vi "excelDispatchNew.vi"() -> ()   [LabVIEW 2012]
uses:
  <vilib>/Utility/NIReport.llb/NI_report.lvclass
  Global1.vi
  <vilib>/addons/database/Connection.llb/DB Tools Open Connec (Path).vi
  <vilib>/addons/_office/excel.llb/Excel Get Data (str).vi
  <vilib>/Utility/NIReport.llb/Excel/NI_Excel.lvclass
  <vilib>/addons/_office/NI_ReportGenerationToolkit.lvlib
  <vilib>/addons/database/NI_Database_API.lvlib
panel:
  out "filenames":string[](array[string])
  out "appended path":path
  out "x+y":i32
  out "error out 3":errorcluster
  out "String 2":string
  out "row":i32
  out "error out":errorcluster
  in  "start (0, 0)":cluster{"start row":i32, "start column":i32}
  out "error out 4":errorcluster
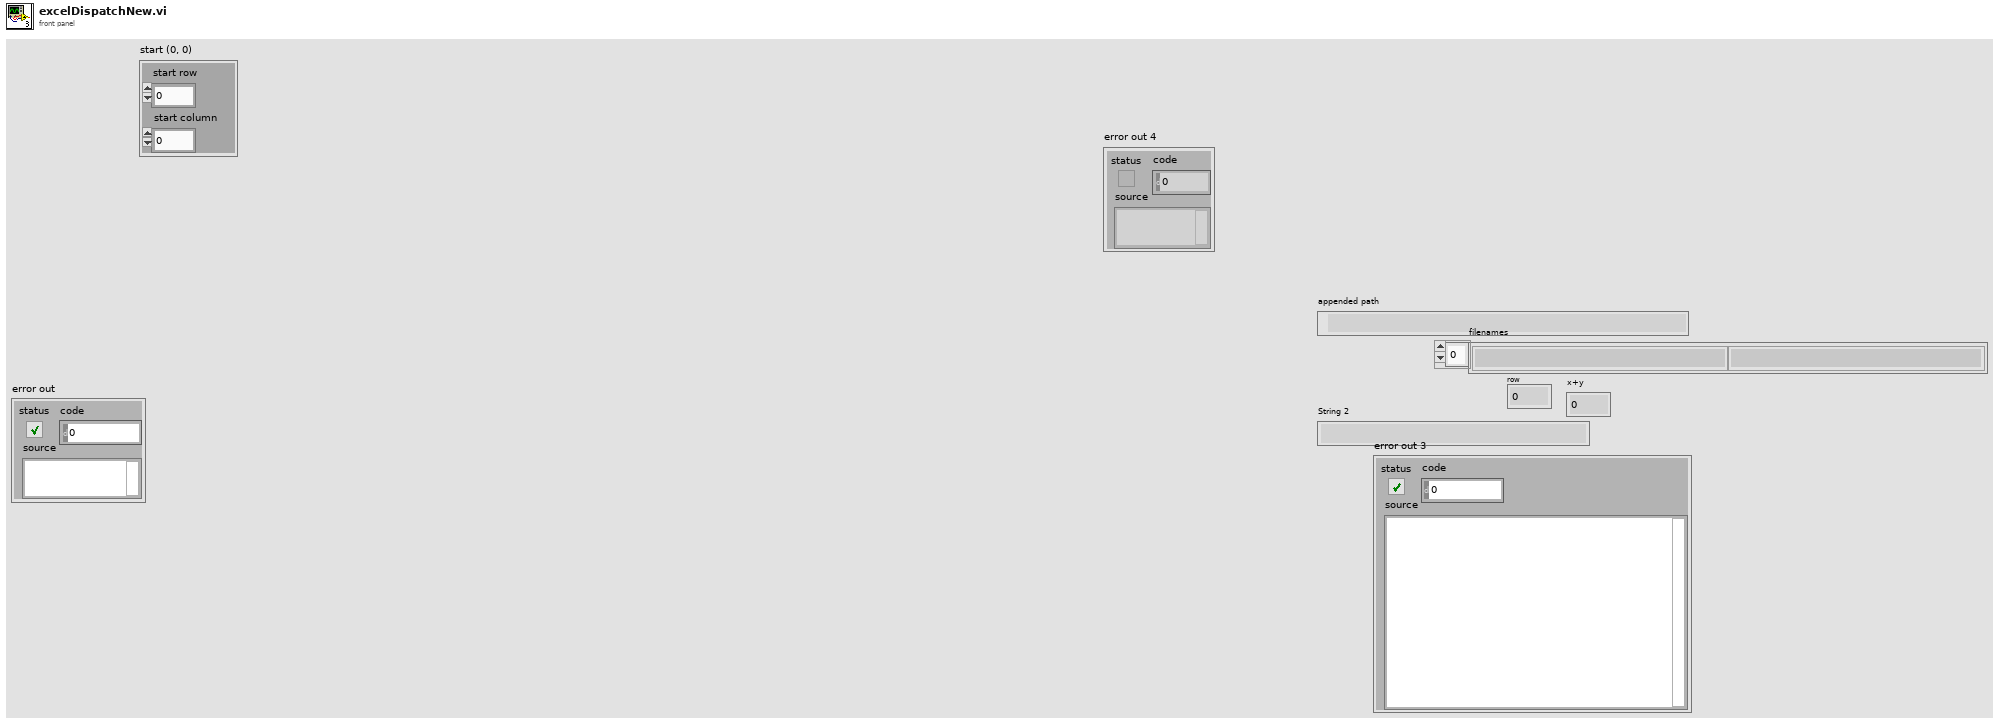
[diagram p1: front panel]
types:
  T1 = enum16{"Standard Report", "HTML", "Word", "Excel"}
  T2 = typedef "NI_Database_API.lvlib/Conn ObjectReference.ctl" = refnum<k1>
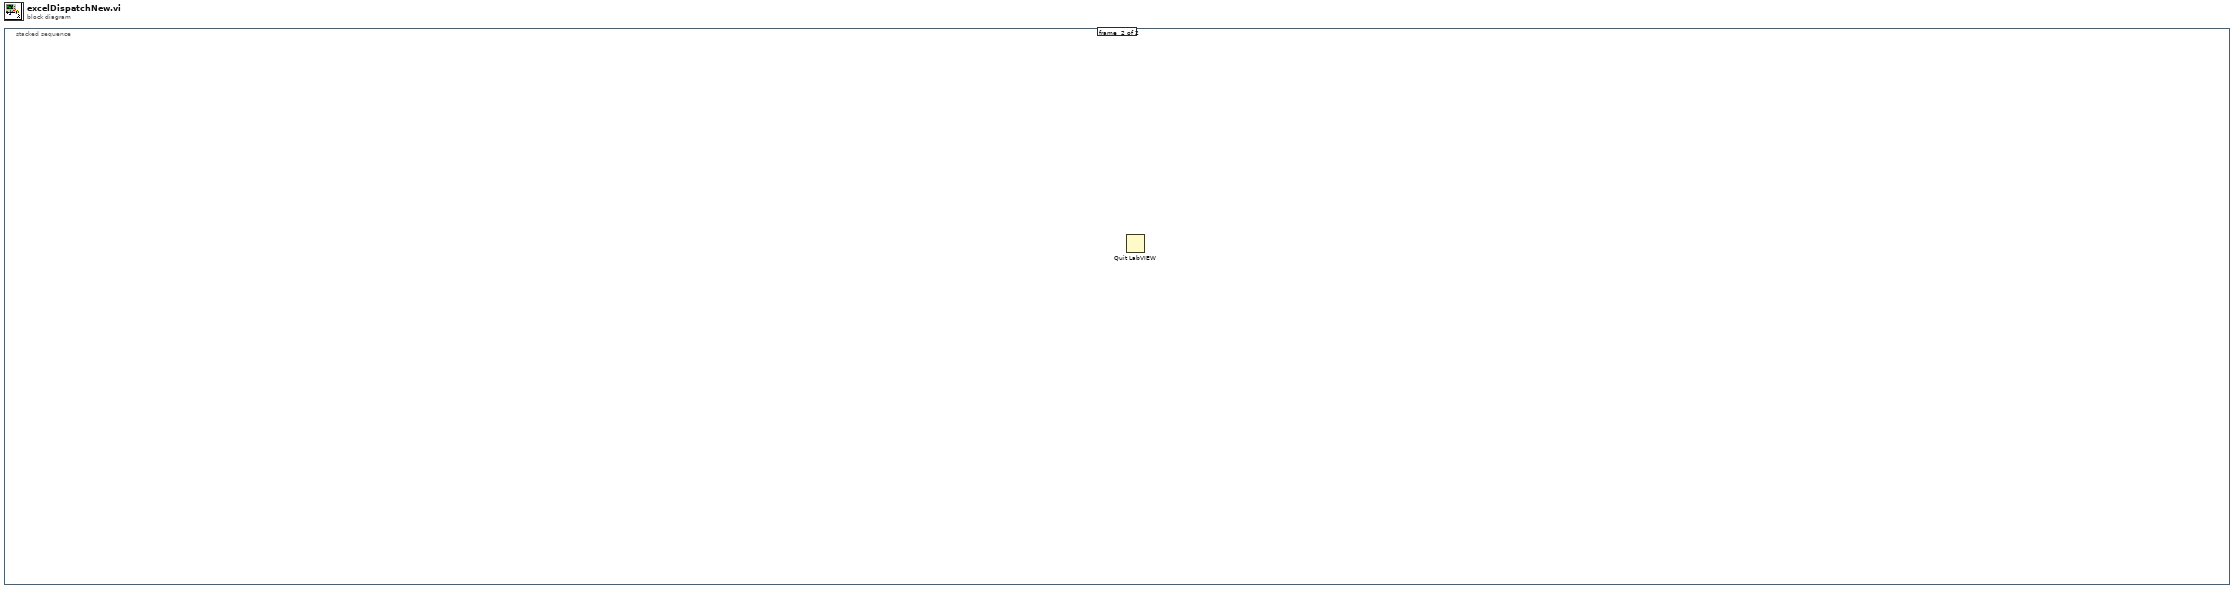
[diagram p0: block diagram]
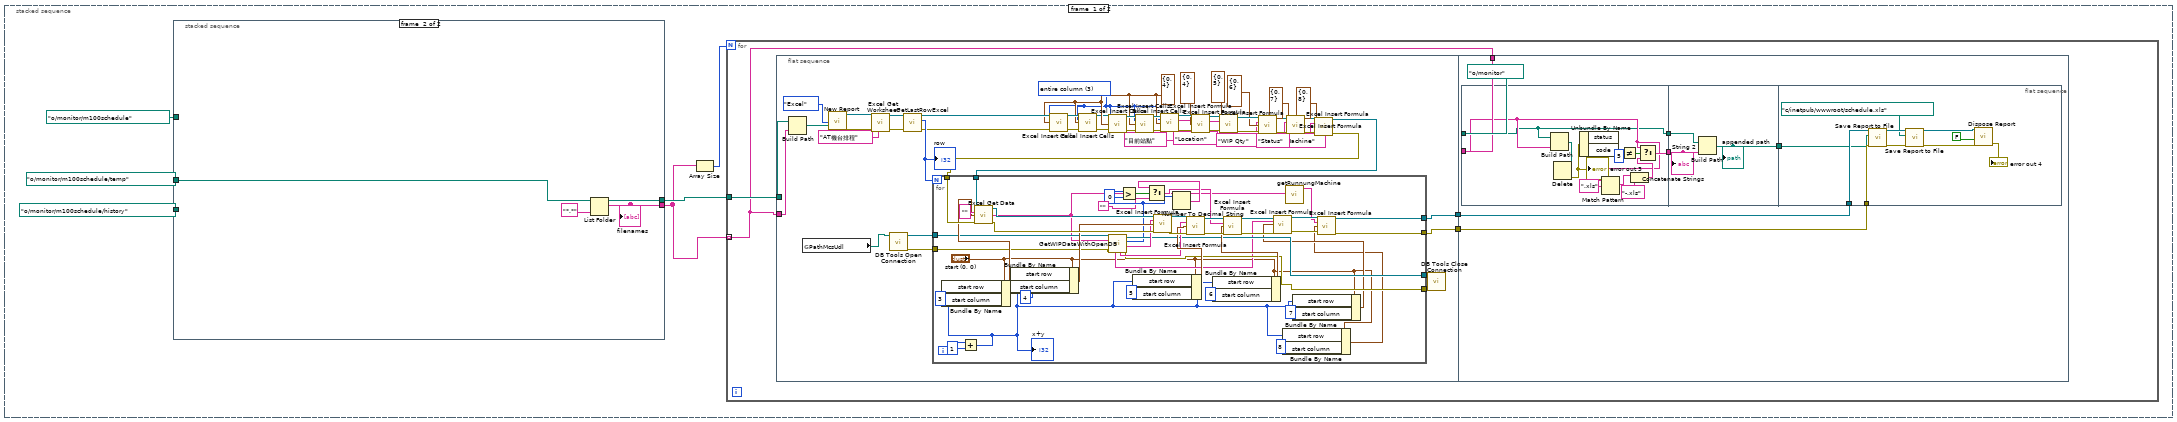
[diagram p2: hidden frame]
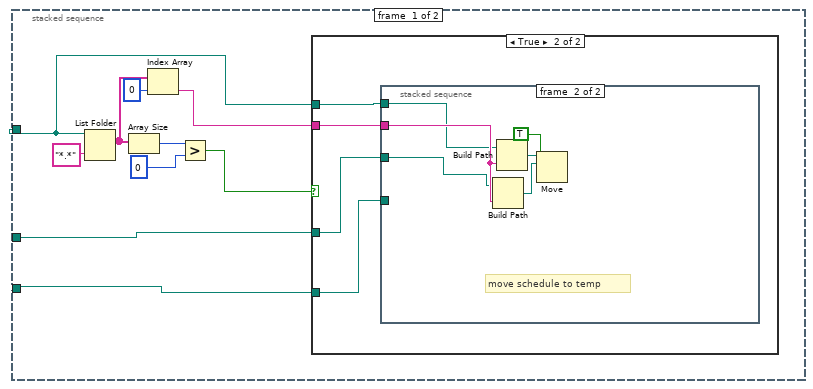
[diagram p3: hidden frame]
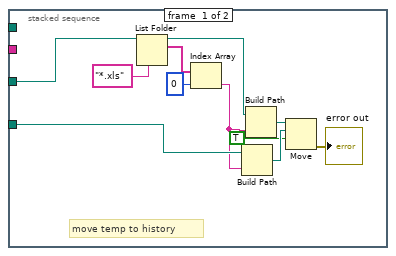
[diagram p5: hidden frame]
diagram:
  n1 = stacked-sequence {
    frame #0 {
      n2 = stacked-sequence {
        tunnel: path "o:/monitor/m100schedule/temp" ("path") -> [w7 w40]
        tunnel: [_ w39] -> w5
        tunnel: path "o:/monitor/m100schedule" ("path") -> [w9 _]
        tunnel: path "o:/monitor/m100schedule/history" ("path") -> [w8 _]
        tunnel: [_ w38] -> w1
        frame #0 {
          n3 = List Folder(path=w9, pattern="*.*") -> (filenames=w13:string[])  [unwired: 2 in, 3 out]
          n4 = Array Size(array=w13) -> (size(s)=w15:i32)
          n5 = Index Array(array=w13, index=0) -> (element=w11:string)
          n6 = Greater?(x=w15, y=0) -> (0:w12:bool)
          n7 = case shown="True" w12 {
            tunnel: w7 -> [_ w20]
            tunnel: w8 -> [_ w19]
            tunnel: w9 -> [_ w18]
            tunnel: w11 -> [_ w17]
            frame False {
            }
            frame True {
              n8 = stacked-sequence {
                tunnel: w20 -> [w27 w33]
                tunnel: w19 -> [w30 _]
                tunnel: w18 -> [_ w34]
                tunnel: w17 -> [_ w35]
                frame #0 {
                  # "move temp to history"
                  n9 = List Folder(path=w27, pattern="*.xls") -> (path out=w25:path, filenames=w24:string[])  [unwired: 2 in, 2 out]
                  n10 = Index Array(array=w24, index=0) -> (element=w22:string)
                  n11 = Build Path(base path=w30, name or relative path=w22) -> (appended path=w29:path)
                  n12 = Build Path(base path=w25, name or relative path=w22) -> (appended path=w31:path)
                  n13 = Move(source path=w31, 9:TRUE ("overwrite (F)"), 10:w29) -> (error out=→"error out":errorcluster)  [unwired: 2 in, 2 out]
                }
                frame #1 {
                  # "move schedule to temp"
                  n14 = Build Path(base path=w33, name or relative path=w35) -> (appended path=w36:path)
                  n15 = Build Path(base path=w34, name or relative path=w35) -> (appended path=w37:path)
                  n16 = Move(source path=w37, 9:TRUE ("overwrite (F)"), 10:w36) -> ()  [unwired: 2 in, 3 out]
                }
              }
            }
          }
        }
        frame #1 {
          n17 = List Folder(path=w40, pattern="*.*") -> (path out=w39:path, filenames=w38:string[])  [unwired: 2 in, 2 out]
          "filenames" <- w38
        }
      }
      n18 = Array Size(array=w1) -> (size(s)=w2:i32)
      n19 = for {
        N: w2 -> [_]
        tunnel: w5 -> [w45]
        tunnel: w1 -> [w42] mode=indexing
        n20 = flat-sequence {
          tunnel: w45 -> [w96]
          tunnel: w42 -> [w95]
          tunnel: [w69] -> w44
          tunnel: [w49] -> w43
          tunnel: w44 -> [w144]
          tunnel: w43 -> [w145]
          tunnel: w42 -> [w146]
          frame #0 {
            w61 = cluster{"row":i32, "column":i32} {"row"=0, "column"=4} ("start (0, 0)")
            w58 = u16 3 items=["shift cells right", "shift cells down", "entire row", "entire column"] ("mode (entire row)")
            n21 = Build Path(base path=w96, name or relative path=w95) -> (appended path=w94:path)
            n22 = global read "Global1.vi" "PathMcsUdl"() -> (w84:path)
            n23 = call <vilib>:"New Report.vi"("report type"=T1."Excel" ("Report Type"), "template (empty)"=w94) -> ("report out"=w92:refnum<class "NI_report.lvclass">, "error out"=w91:errorcluster)  [unwired: 12 in]
            n24 = call <vilib>:"Excel Get Worksheet.vi"("report in"=w92, "error in (no error)"=w91, "name (\"\")"="AT機台排程" ("name (\"\")")) -> ("report out"=w68:refnum<class "NI_report.lvclass">, "error out"=w67:errorcluster)  [unwired: 11 in]
            n25 = call-poly <vilib>:"DB Tools Open Connection.vi"("connection information"=w84) -> ("error out"=w82:errorcluster, "connection reference"=w83:T2)  [unwired: 7 in]
            n26 = call "GetLastRowExcel.vi"("error in (no error)"=w67, "report in"=w68) -> ("error out"=w65:errorcluster, "row"=w66:i32, "report out"=w64:refnum<class "NI_report.lvclass">)  [unwired: 7 in]
            "row" <- w66
            n27 = call <vilib>:"Excel Insert Cells.vi"("report in"=w64, "mode (entire row)"=w58, "start (0, 0)"=w61, "error in (no error)"=w65) -> ("report out"=w63:refnum<class "NI_report.lvclass">, "error out"=w62:errorcluster)  [unwired: 10 in]
            n28 = call <vilib>:"Excel Insert Cells.vi"("report in"=w63, "mode (entire row)"=w58, "start (0, 0)"=w61, "error in (no error)"=w62) -> ("report out"=w60:refnum<class "NI_report.lvclass">, "error out"=w59:errorcluster)  [unwired: 10 in]
            n29 = call <vilib>:"Excel Insert Cells.vi"("report in"=w60, "mode (entire row)"=w58, "start (0, 0)"=w61, "error in (no error)"=w59) -> ("report out"=w90:refnum<class "NI_report.lvclass">, "error out"=w88:errorcluster)  [unwired: 10 in]
            n30 = call <vilib>:"Excel Insert Cells.vi"("report in"=w90, "mode (entire row)"=w58, "start (0, 0)"=w61, "error in (no error)"=w88) -> ("report out"=w89:refnum<class "NI_report.lvclass">, "error out"=w87:errorcluster)  [unwired: 10 in]
            n31 = call <vilib>:"Excel Insert Cells.vi"("report in"=w89, "mode (entire row)"=w58, "start (0, 0)"=w61, "error in (no error)"=w87) -> ("report out"=w81:refnum<class "NI_report.lvclass">, "error out"=w78:errorcluster)  [unwired: 10 in]
            n32 = call <vilib>:"Excel Insert Formula.vi"("report in"=w81, "formula"="目前站點", "start (0, 0)"=cluster{"row":i32, "column":i32} {"row"=0, "column"=4}, "error in (no error)"=w78) -> ("report out"=w80:refnum<class "NI_report.lvclass">, "error out"=w77:errorcluster)  [unwired: 10 in]
            n33 = call <vilib>:"Excel Insert Formula.vi"("report in"=w80, "formula"="Location", "start (0, 0)"=cluster{"row":i32, "column":i32} {"row"=0, "column"=5}, "error in (no error)"=w77) -> ("report out"=w79:refnum<class "NI_report.lvclass">, "error out"=w76:errorcluster)  [unwired: 10 in]
            n34 = call <vilib>:"Excel Insert Formula.vi"("report in"=w79, "formula"="WIP Qty", "start (0, 0)"=cluster{"row":i32, "column":i32} {"row"=0, "column"=6}, "error in (no error)"=w76) -> ("report out"=w57:refnum<class "NI_report.lvclass">, "error out"=w55:errorcluster)  [unwired: 10 in]
            n35 = call <vilib>:"Excel Insert Formula.vi"("report in"=w57, "formula"="Status", "start (0, 0)"=cluster{"row":i32, "column":i32} {"row"=0, "column"=7}, "error in (no error)"=w55) -> ("report out"=w56:refnum<class "NI_report.lvclass">, "error out"=w54:errorcluster)  [unwired: 10 in]
            n36 = call <vilib>:"Excel Insert Formula.vi"("report in"=w56, "formula"="Machine", "start (0, 0)"=cluster{"row":i32, "column":i32} {"row"=0, "column"=8}, "error in (no error)"=w54) -> ("report out"=w52:refnum<class "NI_report.lvclass">, "error out"=w53:errorcluster)  [unwired: 10 in]
            n37 = for {
              N: w66 -> [_]
              tunnel: w52 -> [w142]
              tunnel: w53 -> [w141]
              tunnel: [w105] -> w69
              tunnel: [w123] -> w86
              tunnel: [w122] -> w85
              tunnel: w83 -> [w121]
              tunnel: w82 -> [w120]
              tunnel: [w106] -> w49
              i -> [w113]
              n38 = Add(x=w113, y=1) -> (x+y=w102:i32)
              "x+y" <- w102
              n39 = Bundle By Name(cluster="start (0, 0)", "start row"=w102, "start column"=3) -> (w136:cluster{"start row":i32, "start column":i32})
              n40 = call-poly <vilib>:"Excel Get Data.vi"("report in"=w142, "data type"="", "start (0, 0)"=w136, "error in (no error)"=w141) -> ("report out"=w139:refnum<class "NI_report.lvclass">, "data"=w97:string, "error out"=w138:errorcluster)  [unwired: 9 in]
              n41 = Bundle By Name(cluster="start (0, 0)", "start row"=w102, "start column"=4) -> (w134:cluster{"start row":i32, "start column":i32})
              n42 = call "GetWIPDataWithOpenDB.vi"("error in (no error)"=w120, "Lotno"=w97, "connection reference"=w121) -> ("error out"=w122:errorcluster, "step"=w125:string, "data"=w118:i32, "connection reference 2"=w123:T2, "location"=w124:string, "status"=w103:string)  [unwired: 3 in]
              n43 = Greater?(x=w118, y=0) -> (0:w116:bool)
              n44 = Bundle By Name(cluster="start (0, 0)", "start row"=w102, "start column"=5) -> (w126:cluster{"start row":i32, "start column":i32})
              n45 = call <vilib>:"Excel Insert Formula.vi"("report in"=w139, "formula"=w125, "start (0, 0)"=w134, "error in (no error)"=w138) -> ("report out"=w131:refnum<class "NI_report.lvclass">, "error out"=w128:errorcluster)  [unwired: 10 in]
              n46 = Number To Decimal String(number=w118) -> (decimal integer string=w117:string)  [unwired: 1 in]
              n47 = Select(t=w117, s=w116, f="") -> (s? t:f=w114:string)
              n48 = call <vilib>:"Excel Insert Formula.vi"("report in"=w131, "formula"=w124, "start (0, 0)"=w126, "error in (no error)"=w128) -> ("report out"=w130:refnum<class "NI_report.lvclass">, "error out"=w129:errorcluster)  [unwired: 10 in]
              n49 = Bundle By Name(cluster="start (0, 0)", "start row"=w102, "start column"=6) -> (w127:cluster{"start row":i32, "start column":i32})
              n50 = call <vilib>:"Excel Insert Formula.vi"("report in"=w130, "formula"=w114, "start (0, 0)"=w127, "error in (no error)"=w129) -> ("report out"=w110:refnum<class "NI_report.lvclass">, "error out"=w109:errorcluster)  [unwired: 10 in]
              n51 = Bundle By Name(cluster="start (0, 0)", "start row"=w102, "start column"=8) -> (w100:cluster{"start row":i32, "start column":i32})
              n52 = call "getRunnungMachine.vi"("rc_no"=w97) -> ("machine"=w98:string)  [unwired: 9 in, 1 out]
              n53 = Bundle By Name(cluster="start (0, 0)", "start row"=w102, "start column"=7) -> (w104:cluster{"start row":i32, "start column":i32})
              n54 = call <vilib>:"Excel Insert Formula.vi"("report in"=w110, "formula"=w103, "start (0, 0)"=w104, "error in (no error)"=w109) -> ("report out"=w108:refnum<class "NI_report.lvclass">, "error out"=w107:errorcluster)  [unwired: 10 in]
              n55 = call <vilib>:"Excel Insert Formula.vi"("report in"=w108, "formula"=w98, "start (0, 0)"=w100, "error in (no error)"=w107) -> ("report out"=w106:refnum<class "NI_report.lvclass">, "error out"=w105:errorcluster)  [unwired: 10 in]
            }
            n56 = call <vilib>:"DB Tools Close Connection.vi"("error in (no error)"=w85, "connection reference"=w86) -> ()  [unwired: 5 in, 1 out]
          }
          frame #1 {
            n57 = flat-sequence {
              tunnel: path "o:/monitor" ("base path") -> [w150]
              tunnel: [w150] -> w149
              tunnel: w146 -> [w151]
              tunnel: [w152] -> w148
              tunnel: w149 -> [w164]
              tunnel: w148 -> [w163]
              tunnel: [w162] -> w143
              tunnel: w145 -> [w172]
              tunnel: w144 -> [w171]
              tunnel: w143 -> [w170]
              frame #0 {
                n58 = Build Path(base path=w150, name or relative path=w151) -> (appended path=w161:path)
                n59 = Delete(path (use dialog)=w161) -> (error out=w160:errorcluster)  [unwired: 4 in, 2 out]
                "error out 3" <- w160
                n60 = Unbundle By Name(w160) -> ("code"=w159:i32)  [unwired: 1 out]
                n61 = Match Pattern(string=w151, regular expression=".xls") -> (match substring=w154:string)  [unwired: 1 in, 3 out]
                n62 = Not Equal?(x=w159, y=5) -> (x != y?=w157:bool)
                n63 = Concatenate Strings(w154, "-.xls" ("string")) -> (w155:string)
                n64 = Select(t=w151, s=w157, f=w155) -> (s? t:f=w152:string)
              }
              frame #1 {
                n65 = Build Path(base path=w164, name or relative path=w163) -> (appended path=w162:path)
                "appended path" <- w162
                "String 2" <- w163
              }
              frame #2 {
                n66 = call-dynamic "Save Report to File.vi"("report in"=w172, "report file path"=w170, "error in (no error)"=w171) -> ("report out"=w169:refnum<class "NI_report.lvclass">, "error out"=w167:errorcluster)  [unwired: 11 in]
                n67 = call-dynamic "Save Report to File.vi"("report in"=w169, "report file path"=path "c:/inetpub/wwwroot/schedule.xls", "error in (no error)"=w167) -> ("report out"=w168:refnum<class "NI_report.lvclass">, "error out"=w166:errorcluster)  [unwired: 11 in]
                n68 = call-dynamic "Dispose Report.vi"("report in"=w168, "save changes? (F)"=FALSE, "error in (no error)"=w166) -> ("error out"=→"error out 4":errorcluster)  [unwired: 12 in]
              }
            }
          }
        }
      }
    }
    frame #1 {
      n69 = Quit LabVIEW() -> ()  [unwired: 1 in]
    }
  }
